vi "RT Obtain Queue.vi"(8 "error in":errorcluster) -> (0 "error out":errorcluster, 3 "Queue ref":T1)   [LabVIEW 2022 SP3]
uses:
  RT Controls/RT All Queue.ctl
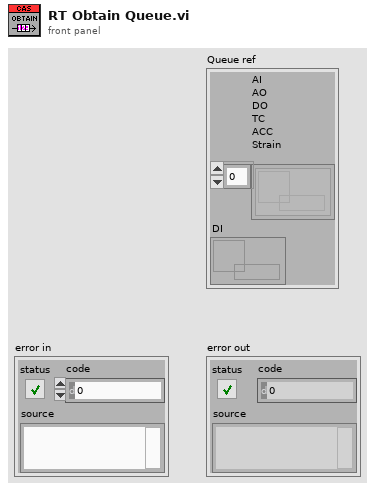
[diagram p1: front panel]
types:
  T1 = typedef "RT All Queue.ctl" = cluster{"AI\nAO\nDO\nTC\nACC\nStrain":refnum<queue>[], "DI":refnum<queue>}
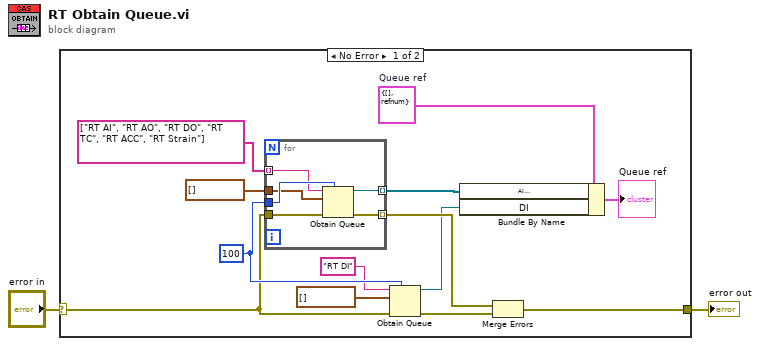
[diagram p0: block diagram]
diagram:
  n1 = case shown="No Error" "error in" {
    selector: "error in" -> [w9 w22]
    tunnel: [w7 w22] -> w1
    frame No Error {
      w6 = T1 {"AI\nAO\nDO\nTC\nACC\nStrain"=[], "DI"=refnum}  # Queue ref
      w12 = 100 ("max queue size (-1, unlimited)")
      n2 = for {
        tunnel: w12 -> [w21]
        tunnel: string[] ["RT AI", "RT AO", "RT DO", "RT TC", "RT ACC", "RT Strain"] ("name (unnamed)") -> [w20] mode=indexing
        tunnel: waveform(dbl)[] [] ("Waveform") -> [w19]
        tunnel: w9 -> [w18]
        tunnel: [w17] -> w13 mode=indexing
        tunnel: [w16] -> w5 mode=indexing
        n3 = Obtain Queue(max queue size (-1, unlimited)=w21, name (unnamed)=w20, element data type=w19, error in (no error)=w18) -> (queue out=w16:refnum<queue>, error out=w17:errorcluster)  [unwired: 1 in, 1 out]
      }
      n4 = Obtain Queue(max queue size (-1, unlimited)=w12, name (unnamed)="RT DI", element data type=digitalwaveform[] [] ("output waveform"), error in (no error)=w9) -> (queue out=w4:refnum<queue>, error out=w8:errorcluster)  [unwired: 1 in, 1 out]
      n5 = Bundle By Name(cluster=w6, "AI\nAO\nDO\nTC\nACC\nStrain"=w5, "DI"=w4) -> (→"Queue ref":T1)
      n6 = Merge Errors(w13, w8) -> (w7:errorcluster)
    }
    frame Error {
    }
  }
  "error out" <- w1
